vi "Read configuration.vi"(8 "error in":errorcluster, 11 "JSON_RPC_Interface editor node in":refnum<class "JSON_RPC_Interface editor node.lvclass">) -> (0 "error out":errorcluster, 2 "configuration":refnum<class "NISE_CEF_serializable configuration.lvclass">, 3 "JSON_RPC_Interface editor node out":refnum<class "JSON_RPC_Interface editor node.lvclass">)   [LabVIEW 2018, in "JSON_RPC_Interface editor node.lvclass"]
uses:
  JSON_RPC_Interface editor node.lvclass
  <vilib>/NI/Configuration Framework/serializable configuration/NISE_CEF_serializable configuration.lvclass
  JSON_RPC_Interface editor node.lvclass/JSON_RPC_Interface editor node.ctl
  module/configuration/JSON_RPC_Interface configuration.lvclass
  C:/Program Files (x86)/National Instruments/LabVIEW 2018/vi.lib/NI/Configuration Framework/serializable configuration/NISE_CEF_serializable configuration.lvclass
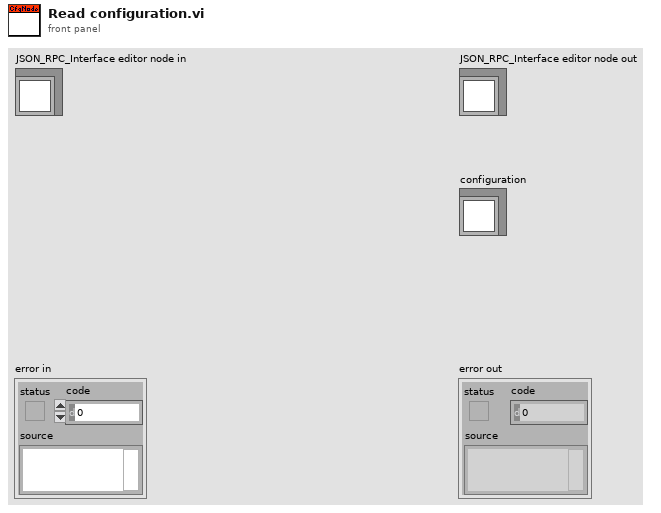
[diagram p1: front panel]
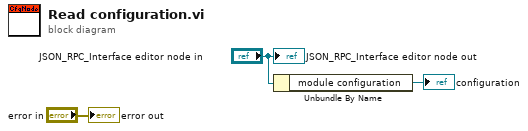
[diagram p0: block diagram]
diagram:
  n1 = Unbundle By Name("JSON_RPC_Interface editor node in") -> ("module configuration"=→"configuration":refnum<class "JSON_RPC_Interface configuration.lvclass">)
  "error out" <- "error in"
  "JSON_RPC_Interface editor node out" <- "JSON_RPC_Interface editor node in"
